vi "Initialize From Settings.vi"(8 "error in (no error)":errorcluster, 10 "settings":cluster{"key":string, "value":string}[](array[cluster]), 11 "UDP Thread Configuration in":refnum<class "UDP Thread Configuration.lvclass">) -> (0 "error out":errorcluster, 3 "UDP Thread Configuration out":refnum<class "UDP Thread Configuration.lvclass">)   [LabVIEW 2020, in "UDP.lvlib" / "UDP Thread Configuration.lvclass"]
uses:
  UDP Thread Configuration.lvclass
  UDP Thread Configuration.lvclass/UDP Thread Configuration.ctl
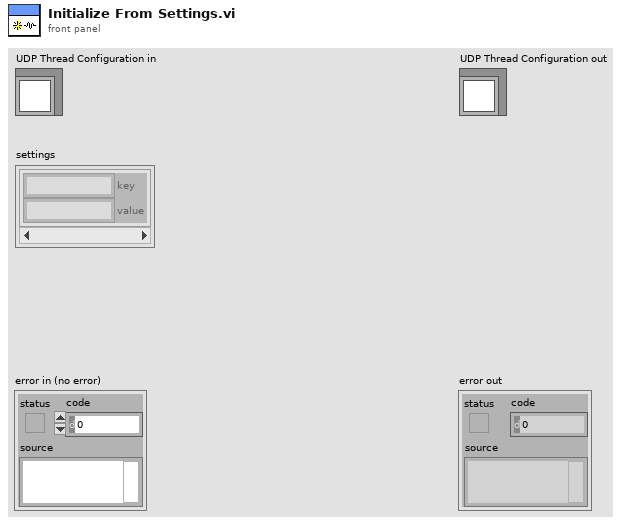
[diagram p1: front panel]
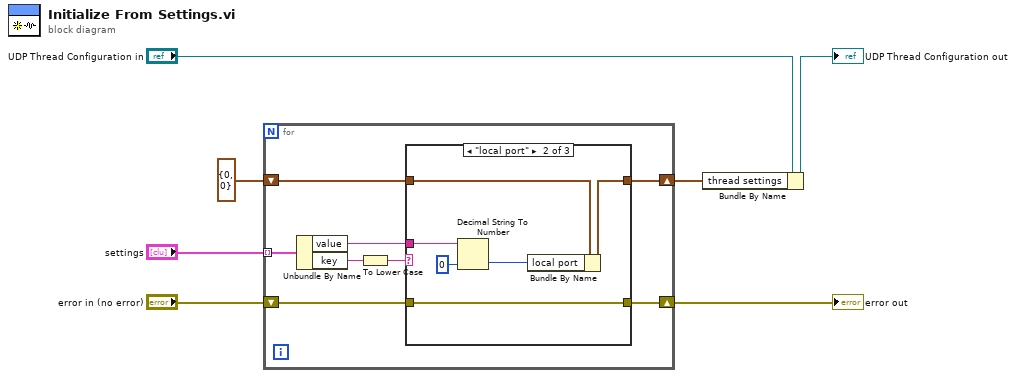
[diagram p0: block diagram]
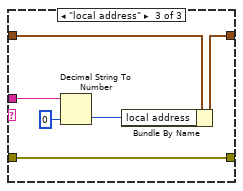
[diagram p3: hidden frame]
diagram:
  n1 = for {
    shift-right: [w8] -> w3
    shift-left: "error in (no error)" -> [w14]
    shift-right: [w10] -> w1
    shift-left: cluster{"local port":u16, "local address":u32} {"local port"=0, "local address"=0} ("thread settings") -> [w11]
    tunnel: "settings" -> [w15] mode=indexing
    n2 = Unbundle By Name(w15) -> ("value"=w12:string, "key"=w13:string)
    n3 = To Lower Case(string=w13) -> (all lower case string=w9:string)
    n4 = case shown="\"local port\"" w9 {
      tunnel: w14 -> [w16 w21 w27]
      tunnel: w12 -> [_ w20 w25]
      tunnel: w11 -> [w17 w23 w29]
      tunnel: [w17 w22 w28] -> w10
      tunnel: [w16 w21 w27] -> w8
      frame Default {
        # "Unknown Setting."
      }
      frame "local port" {
        n5 = Decimal String To Number(string=w20, default (0L)=u16 0 ("default (0 I32)")) -> (number=w19:u16)  [unwired: 1 in, 1 out]
        n6 = Bundle By Name(cluster=w23, "local port"=w19) -> (w22:cluster{"local port":u16, "local address":u32})
      }
      frame "local address" {
        n7 = Decimal String To Number(string=w25, default (0L)=u32 0 ("default (0 I32)")) -> (number=w24:u32)  [unwired: 1 in, 1 out]
        n8 = Bundle By Name(cluster=w29, "local address"=w24) -> (w28:cluster{"local port":u16, "local address":u32})
      }
    }
  }
  "error out" <- w3
  n9 = Bundle By Name(cluster="UDP Thread Configuration in", "thread settings"=w1) -> (→"UDP Thread Configuration out":refnum<class "UDP Thread Configuration.lvclass">)
